vi "Handle Error.vi"(8 "error in (no error)":errorcluster, 11 "Measure Object in":refnum<class "Application Controller.lvclass">) -> (0 "error out":errorcluster, 2 "stop actor?":bool=TRUE, 3 "Measure Object out":refnum<class "Application Controller.lvclass">)   [LabVIEW 2019, in "Application Controller.lvclass"]
doc: "(<B>Filename</B>: Actor Framework.lvlib:Actor.lvclass:Handle Error.vi)\n\nDefines how the actor handles an error that occurred while processing a message. By default, this method does nothing except stop the actor."
uses:
  Application Controller.lvclass
  C:/Program Files/National Instruments/LabVIEW 2019/vi.lib/ActorFramework/Actor/Actor.lvclass
  <vilib>/ActorFramework/Actor/Actor.lvclass/Actor.ctl
  Application Controller Messages/Display Error Msg/Display Error Msg.lvclass/Display Error Msg.ctl
  <vilib>/ActorFramework/Message Enqueuer/Message Enqueuer.lvclass/Message Enqueuer.ctl
  <vilib>/ActorFramework/Message Enqueuer/Enqueue.vi
  <vilib>/ActorFramework/Message Enqueuer/Init from Existing Queue.vi
  Application Controller Messages/Display Error Msg/Display Error Msg.lvclass
  C:/Program Files/National Instruments/LabVIEW 2019/vi.lib/ActorFramework/Message/Message.lvclass
  <vilib>/ActorFramework/Stop Msg/Stop Msg.lvclass
  <vilib>/ActorFramework/Message Priority Queue/Priority Enqueue.vi
  Process Controller/Process Controller.lvclass
  <vilib>/ActorFramework/Message Enqueuer/Message Enqueuer.lvclass
  <vilib>/ActorFramework/Actor/Actor.lvclass
  C:/GitHub/LabActor/Controllers/Process Controller/Process Controller.lvclass
  C:/GitHub/LabActor/Worker/Worker.lvclass
  C:/GitHub/LabActor/Template Module/Template Module.lvclass
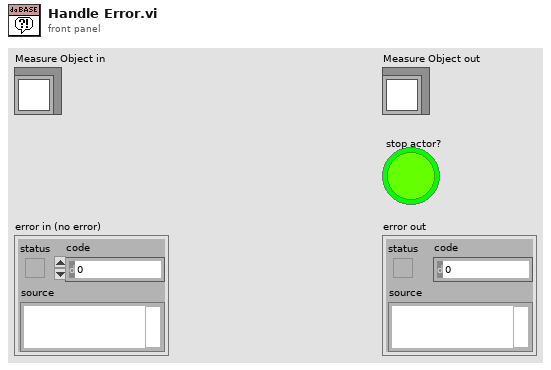
[diagram p1: front panel]
types:
  T1 = typedef "LabActor Error.ctl" = cluster{"Time":string, "Message":string, "Source":string, "Code":i32, "Error?":bool, "Module":string}
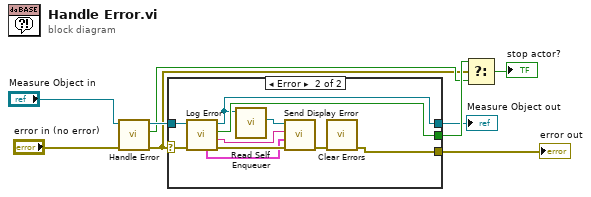
[diagram p0: block diagram]
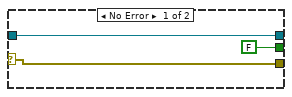
[diagram p2: hidden frame]
diagram:
  n1 = call-parent "Handle Error.vi"("error in (no error)"="error in (no error)", "Measure Object in"="Measure Object in") -> ("error out"=w2:errorcluster, "stop actor?"=w5:bool, "Measure Object out"=w7:refnum<class "Application Controller.lvclass">)  [unwired: 7 in]
  n2 = case shown="Error" w2 {
    selector: w2 -> [w10 w17]
    tunnel: w7 -> [w11 w22]
    tunnel: [FALSE w21] -> w6
    tunnel: [w11 w18] -> w3
    tunnel: [w10 w13] -> w1
    frame No Error {
    }
    frame Error {
      n3 = call-dynamic "Log Error.vi"("error in (no error)"=w17, "Da Base in"=w22) -> ("error out"=w20:errorcluster, "Error message"=w19:string, "stop actor?"=w21:bool, "Da Base out"=w18:refnum<class "Application Controller.lvclass">, "LabActor Error"=w16:T1)  [unwired: 5 in]
      n4 = call <vilib>:"Read Self Enqueuer.vi"("Actor"=w18) -> ("Self Enqueuer"=w15:refnum<class "Message Enqueuer.lvclass">)  [unwired: 10 in]
      n5 = call "Send Display Error.vi"("error in (no error)"=w20, "LabActor Error"=w16, "Error message"=w19, "Message Enqueuer"=w15) -> ("error out"=w14:errorcluster)  [unwired: 6 in, 1 out]
      n6 = call <vilib>:"Clear Errors.vi"("error in (no error)"=w14) -> ("error out"=w13:errorcluster)  [unwired: 5 in, 1 out]
    }
  }
  "Measure Object out" <- w3
  "error out" <- w1
  n7 = Select(t=w6, s=w2, f=w5) -> (s? t:f=→"stop actor?":bool)
